vi "用户登陆.vi"() -> (0 "退出":bool, 1 "权限out":i32, 2 "用户名out":string, 3 "用户信息out":string[][](array[string]) caption="所有行")   [LabVIEW 2020]
uses:
  <vilib>/Utility/file.llb/Read Delimited Spreadsheet (string).vi
panel:
  out "权限":string
  in  "Btn_Exit":bool
  in  "Btn_Confirm":bool
  in  "密码":string
  in  "用户名":string(combo)
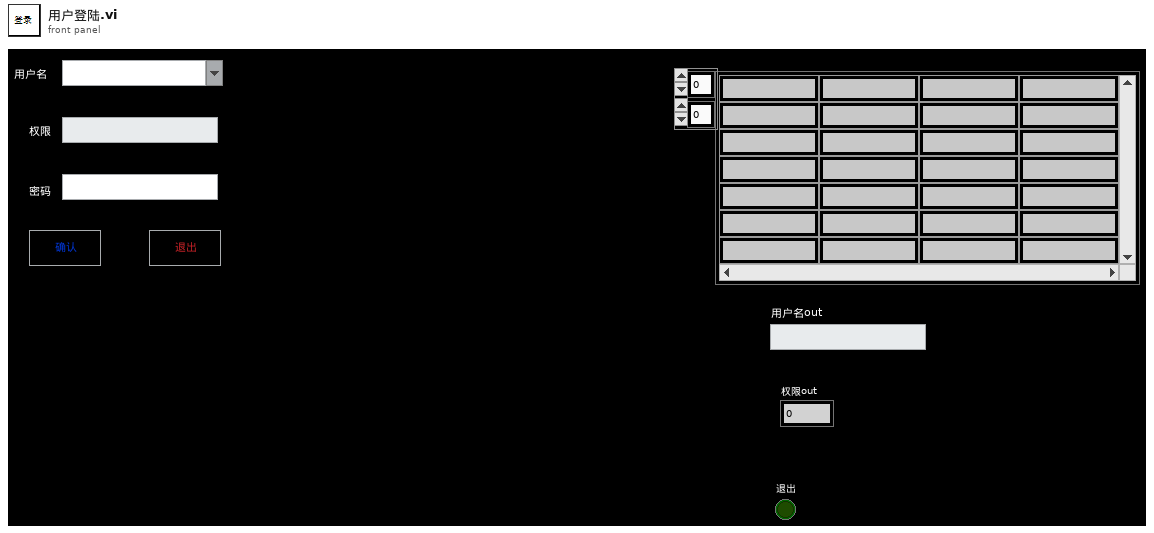
[diagram p1: front panel]
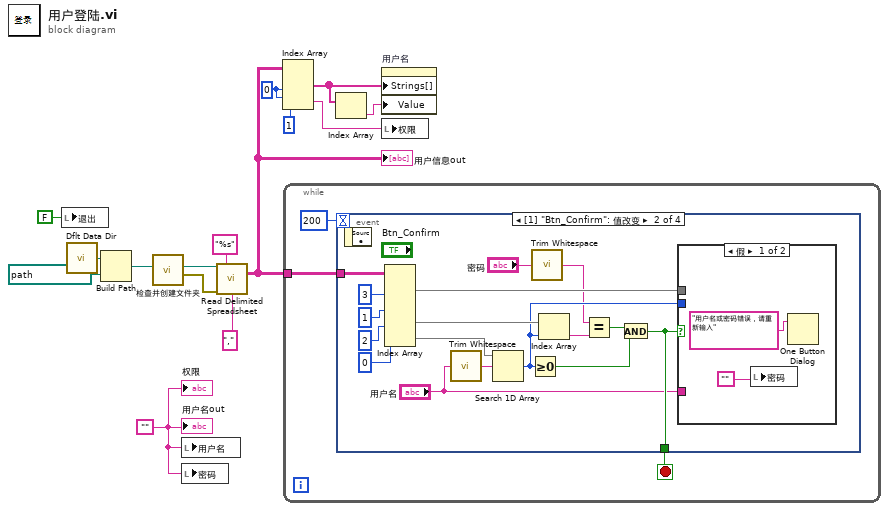
[diagram p0: block diagram]
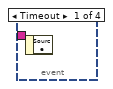
[diagram p2: hidden frame]
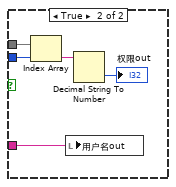
[diagram p3: hidden frame]
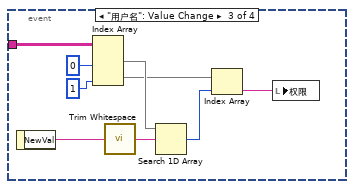
[diagram p4: hidden frame]
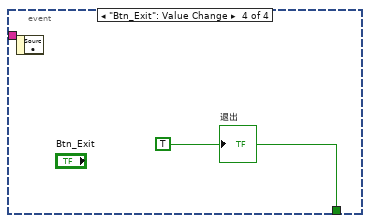
[diagram p5: hidden frame]
diagram:
  w1 = 0 ("禁用的索引 (列)")
  w7 = ""
  n1 = local write "退出"(FALSE ("退出")) -> ()
  n2 = call <vilib>:"Dflt Data Dir.vi"() -> ("App:Default Data Directory"=w14:path)
  n3 = Build Path(base path=w14, name or relative path=path "用户管理.csv" ("名称或相对路径")) -> (appended path=w10:path)
  n4 = call "检查并创建文件夹.vi"("路径in"=w10) -> ("error out"=w8:errorcluster, "dup path"=w9:path)  [unwired: 9 in]
  n5 = local write "用户名"(w7) -> ()
  n6 = local write "密码"(w7) -> ()
  n7 = call-poly <vilib>:"Read Delimited Spreadsheet.vi"("file path (dialog if empty)"=w9, "format (%s)"="%s", "error in (no error)"=w8, "delimiter (\\t)"="," ("delimiter (\\t)")) -> ("all rows"=w6:string[][])  [unwired: 6 in, 5 out]
  "用户信息out" <- w6
  n8 = Index Array(array=w6, index (col) #1=w1, index (row) #2=w1, index (col) #2=1 ("禁用的索引 (列)")) -> (element #1=w5:string[], element #2=w2:string)  [unwired: 1 in]
  n9 = while {
    tunnel: w6 -> [w17]
    stop <- w16 stop-if-true
    n10 = event shown="[1] \"Btn_Confirm\": 值改变" {
      selector: _ -> [_ _ _ _]
      dyn-events: _ -> [_ _ _ _]
      timeout: 200 -> [_ _ _ _]
      tunnel: w17 -> [_ w35 w49 _]
      tunnel: [_ w25 _ w52] -> w16
      event Timeout {
        n11 = event-data() -> ()  [unwired: 1 in, 1 out]
      }
      event "Btn_Confirm": Value Change {
        n12 = event-data() -> ()  [unwired: 1 in, 1 out]
        n13 = Index Array(array=w35, index (col) #1=3 ("禁用的索引 (列)"), index (col) #2=1 ("禁用的索引 (列)"), index (col) #3=2 ("禁用的索引 (列)"), index (col) #4=0 ("禁用的索引 (列)")) -> (element #1=w26:string[], element #3=w24:string[], element #4=w29:string[])  [unwired: 4 in, 1 out]
        n14 = call <vilib>:"Trim Whitespace.vi"("string"="用户名") -> ("trimmed string"=w28:string)  [unwired: 1 in]
        n15 = Search 1D Array(1D array=w29, element=w28) -> (index of element=w23:i32)  [unwired: 1 in]
        n16 = Greater Or Equal To 0?(x=w23) -> (x >= 0?=w27:bool)
        n17 = call <vilib>:"Trim Whitespace.vi"("string"="密码") -> ("trimmed string"=w20:string)  [unwired: 1 in]
        n18 = Index Array(array=w24, index=w23) -> (element=w22:string)
        n19 = Equal?(x=w20, y=w22) -> (x = y?=w21:bool)
        n20 = And(x=w21, y=w27) -> (x .and. y?=w25:bool)
        n21 = case shown="假" w25 {
          tunnel: w26 -> [_ w42]
          tunnel: w23 -> [_ w41]
          tunnel: "用户名" -> [_ w38]
          frame False {
            n22 = local write "密码"("") -> ()
            n23 = One Button Dialog(message="用户名或密码错误，请重新输入" ("消息")) -> ()  [unwired: 1 in, 1 out]
          }
          frame True {
            n24 = Index Array(array=w42, index=w41) -> (element=w40:string)
            n25 = local write "用户名out"(w38) -> ()
            n26 = Decimal String To Number(string=w40) -> (number=→"权限out":i32)  [unwired: 2 in, 1 out]
          }
        }
      }
      event "用户名": Value Change {
        n27 = event-data() -> ("NewVal"=w47:string)  [unwired: 1 in]
        n28 = Index Array(array=w49, index (col) #1=0 ("禁用的索引 (列)"), index (col) #2=1 ("禁用的索引 (列)")) -> (element #1=w46:string[], element #2=w45:string[])  [unwired: 2 in]
        n29 = call <vilib>:"Trim Whitespace.vi"("string"=w47) -> ("trimmed string"=w48:string)  [unwired: 1 in]
        n30 = Search 1D Array(1D array=w46, element=w48) -> (index of element=w44:i32)  [unwired: 1 in]
        n31 = Index Array(array=w45, index=w44) -> (element=w43:string)
        n32 = local write "权限"(w43) -> ()
      }
      event "Btn_Exit": Value Change {
        w52 = TRUE ("退出")
        n33 = event-data() -> ()  [unwired: 1 in, 1 out]
        "退出" <- w52
      }
    }
  }
  n34 = Index Array(array=w5) -> (element=w3:string)  [unwired: 1 in]
  n35 = property on="用户名" class="CmbBox"("Strings[]"=w5, "Value"=w3) -> ()  [unwired: 2 in, 2 out]
  n36 = local write "权限"(w2) -> ()
  "用户名out" <- w7
  "权限" <- w7
